vi "acq.Batch.vi"(6 "# Acq in":u16, 7 "DVR":T1, 8 "error in":errorcluster, 11 "cam in":refnum<class "camera.lvclass">) -> (0 "error out":errorcluster, 1 "PL":u16[][](array[numeric]), 2 "IL":u16[][](array[numeric]), 4 "acq time":dbl)   [LabVIEW 2020]
uses:
  c5544233-71f3-4b66-846b-1f2d698a5cd2.vi
  camera/camera.lvclass
  _controls/mode.ctl
  _controls/data.ref.ctl
  _controls/data.ctl
  _controls/state.ctl
  _controls/data.vars.ctl
  _controls/flip.ctl
  <vilib>/vision/Image Controls.llb/IMAQ Image.ctl
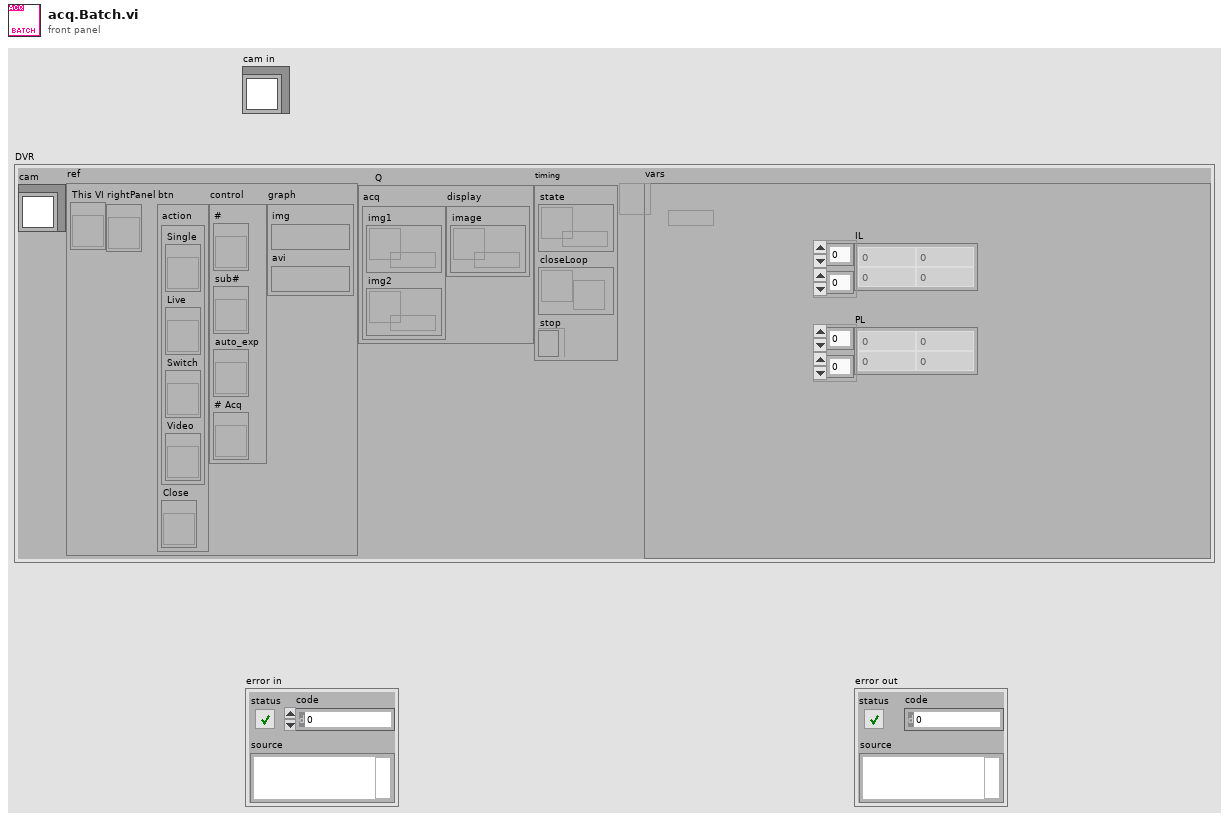
[diagram p1: front panel]
types:
  T1 = typedef "data.ctl" = cluster{"cam":refnum<class "camera.lvclass">, "ref":T2, "Q":cluster{"acq":cluster{"img1":refnum<queue>, "img2":refnum<queue>}, "display":cluster{"image":refnum<queue>}}, "timing":cluster{"state":refnum<queue>, "closeLoop":refnum<notifier>, "stop":refnum<k4>}, "vars":refnum<data-value>}
  T2 = typedef "data.ref.ctl" = cluster{"This VI":refnum<vi>, "rightPanel":refnum<vi>, "btn":cluster{"action":cluster{"Single":refnum<vi>, "Live":refnum<vi>, "Switch":refnum<vi>, "Video":refnum<vi>}, "Close":refnum<vi>}, "control":cluster{"#":refnum<vi>, "sub#":refnum<vi>, "auto_exp":refnum<vi>, "# Acq":refnum<vi>}, "graph":cluster{"img":T3, "avi":T3}}
  T3 = typedef "IMAQ Image.ctl" = refnum<image>
  T4 = typedef "mode.ctl" = enum16{"PL", "EL"}
  T5 = typedef "path.ctl" = cluster{"light":path, "name":string, "full":path}
  T6 = typedef "data.vars.ctl" = cluster{"save":cluster{"base_folder":cluster{"Folder":path, "tif":bool, "jpg":bool}, "module":string, "#":u32, "sub#":u8, "save.op":enum16{"Full", "Light"}, "same?":bool, "Shift":enum16{"Single", "Leapfrog"}, "jpg?":bool, "flip":T7}, "acq":cluster{"# Acq":u16, "rotate":bool, "FPS":dbl}, "calib.manual":cluster{"BG":cluster{"Image":u16[][], "enabled?":bool}, "FF":cluster{"Image":u16[][], "enabled?":bool}}}
  T7 = typedef "flip.ctl" = cluster{"x":bool, "y":bool}
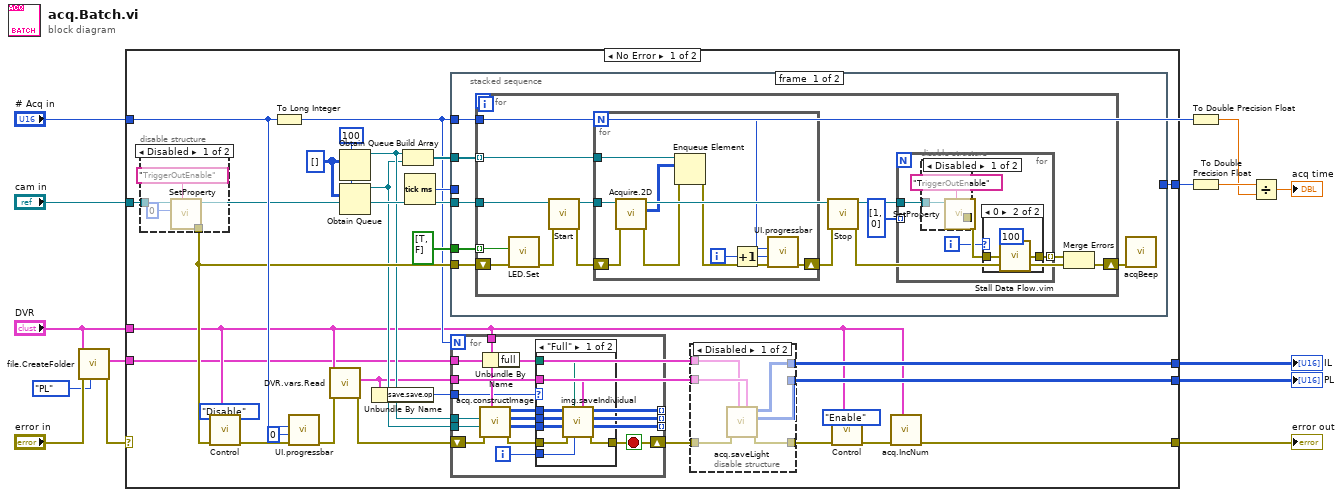
[diagram p0: block diagram]
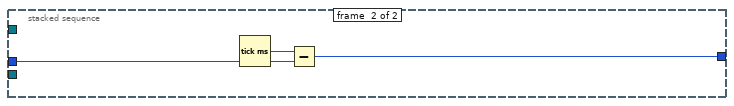
[diagram p6: hidden frame]
diagram:
  n1 = call "file.CreateFolder.vi"("mode"=mode."PL", "error in"="error in", "DVR"="DVR") -> ("error out"=w12:errorcluster, "path"=w9:T5)  [unwired: 7 in]
  n2 = case shown="No Error" w12 {
    selector: w12 -> [_ w118]
    tunnel: "cam in" -> [w31 _]
    tunnel: "# Acq in" -> [w42 _]
    tunnel: [w41 _] -> w13
    tunnel: [w27 w118] -> w2
    tunnel: "DVR" -> [w18 _]
    tunnel: [w25 _] -> w11
    tunnel: [w24 _] -> w10
    tunnel: w9 -> [w15 _]
    frame No Error {
      w36 = u16[][] [] ("buffer")
      w39 = 100 ("max queue size (-1, unlimited)")
      n3 = disable-structure shown="Disabled" {
        disable-tunnel: w31 -> [w52 _]
        disable-tunnel: [w51 _] -> w30
        frame Disabled {
          n4 = call-dynamic "SetProperty.vi"("Property"="TriggerOutEnable" ("pPrp"), "Value"=0 ("lValue"), "camera.nit in"=w52) -> ("error out"=w51:errorcluster)  [unwired: 8 in]
        }
        frame Enabled {
        }
      }
      n5 = call "Control.vi"("mode"=enum16{"Enable", "Disable"}."Disable", "DVR"=w18, "error in"=w30) -> ("error out"=w33:errorcluster)  [unwired: 8 in]
      n6 = To Long Integer(number=w42) -> (32bit integer=w19:i32)
      n7 = call "UI.progressbar.vi"("error in"=w33, "Value"=u8 0, "Maximum"=w42) -> ("error out"=w32:errorcluster)  [unwired: 8 in]
      n8 = call "DVR.vars.Read.vi"("error in"=w32, "DVR.state"=w18) -> ("error out"=w23:errorcluster, "vars"=w17:T6)  [unwired: 8 in]
      n9 = Obtain Queue(max queue size (-1, unlimited)=w39, element data type=w36) -> (queue out=w21:refnum<queue>)  [unwired: 3 in, 2 out]
      n10 = Obtain Queue(max queue size (-1, unlimited)=w39, element data type=w36) -> (queue out=w20:refnum<queue>)  [unwired: 3 in, 2 out]
      n11 = Unbundle By Name(w17) -> ("save.save.op"=w16:enum16{"Full", "Light"})
      n12 = Build Array(w21, w20) -> (w38:refnum<queue>[])
      n13 = Tick Count (ms)() -> (millisecond timer value=w37:u32)
      n14 = stacked-sequence {
        tunnel: bool[] [TRUE, FALSE] -> [w58 _]
        tunnel: w31 -> [w53 _]
        tunnel: w38 -> [w57 _]
        tunnel: w19 -> [w56 _]
        tunnel: w37 -> [_ w93]
        tunnel: [_ w92] -> w41
        tunnel: w30 -> [w55 _]
        frame #0 {
          n15 = for {
            tunnel: w56 -> [w66]
            shift-right: [w64] -> w54
            shift-left: w55 -> [w70]
            tunnel: w58 -> [w69] mode=indexing
            tunnel: w57 -> [w67] mode=indexing
            tunnel: w53 -> [w61]
            n16 = call "LED.Set.vi"("error in"=w70, "LED"=w69) -> ("error out"=w68:errorcluster)  [unwired: 9 in]
            n17 = call-dynamic "Start.vi"("error in"=w68, "camera in"=w61) -> ("error out"=w65:errorcluster)  [unwired: 9 in]
            n18 = for {
              N: w66 -> [w85]
              shift-right: [w83] -> w60
              shift-left: w65 -> [w89]
              tunnel: w61 -> [w90]
              tunnel: w67 -> [w91]
              i -> [w86]
              n19 = call-dynamic "Acquire.2D.vi"("error in"=w89, "camera.nit in"=w90) -> ("error out"=w88:errorcluster, "buffer"=w87:u16[][])  [unwired: 8 in]
              n20 = Enqueue Element(queue=w91, element=w87, error in (no error)=w88) -> (error out=w84:errorcluster)  [unwired: 1 in, 2 out]
              n21 = Increment(x=w86) -> (x+1=w82:i32)
              n22 = call "UI.progressbar.vi"("error in"=w84, "Value"=w82, "Maximum"=w85) -> ("error out"=w83:errorcluster)  [unwired: 8 in]
            }
            n23 = call-dynamic "Stop.vi"("error in"=w60, "camera.nit in"=w61) -> ("error out"=w59:errorcluster)  [unwired: 9 in]
            n24 = for {
              tunnel: w61 -> [w74]
              tunnel: [w72] -> w62 mode=indexing
              tunnel: i32[] [1, 0] ("0, 1") -> [_] mode=indexing
              i -> [w71]
              n25 = disable-structure shown="Disabled" {
                disable-tunnel: w74 -> [w77 _]
                disable-tunnel: [w76 _] -> w73
                frame Disabled {
                  n26 = call-dynamic "SetProperty.vi"("Property"="TriggerOutEnable" ("pPrp"), "camera.nit in"=w77) -> ("error out"=w76:errorcluster)  [unwired: 9 in]
                }
                frame Enabled {
                }
              }
              n27 = case shown="0" w71 {
                tunnel: w73 -> [w78 w81]
                tunnel: [w78 w80] -> w72
                frame Default {
                }
                frame 0 {
                  n28 = call "Stall Data Flow.vim"("value in"=w81, "milliseconds to wait"=u32 100) -> ("value out"=w80:errorcluster)  [unwired: 1 out]
                }
              }
            }
            n29 = Merge Errors(w62, w59) -> (w64:errorcluster)
          }
          n30 = call "acqBeep.vi"("error in"=w54) -> ()  [unwired: 10 in, 1 out]
        }
        frame #1 {
          n31 = Tick Count (ms)() -> (millisecond timer value=w94:u32)
          n32 = Subtract(x=w94, y=w93) -> (x-y=w92:u32)
        }
      }
      n33 = for {
        N: w19 -> [_]
        shift-right: [w98] -> w22
        shift-left: w23 -> [w106]
        tunnel: w20 -> [w107]
        tunnel: w21 -> [w108]
        tunnel: w18 -> [w105]
        tunnel: [w102] -> _ mode=indexing
        tunnel: [w101] -> _ mode=indexing
        tunnel: w17 -> [w100]
        tunnel: [w99] -> _ mode=indexing
        tunnel: w16 -> [w97]
        tunnel: w15 -> [w95]
        i -> [w103]
        stop <- w98 stop-if-true
        n34 = call "acq.constructImage.vi"("DVR"=w105, "error in"=w106, "queue2 in"=w107, "queue1 in"=w108) -> ("error out"=w104:errorcluster, "Dark"=w99:u16[][], "PL"=w101:u16[][], "Bright"=w102:u16[][])  [unwired: 4 in]
        n35 = Unbundle By Name(w95) -> ("full"=w96:path)
        n36 = case shown="\"Full\"" w97 {
          tunnel: w96 -> [w116 _]
          tunnel: w104 -> [w115 w117]
          tunnel: w103 -> [w114 _]
          tunnel: w102 -> [w113 _]
          tunnel: w101 -> [w112 _]
          tunnel: w100 -> [w111 _]
          tunnel: w99 -> [w110 _]
          tunnel: [w109 w117] -> w98
          frame "Full" {
            n37 = call "img.saveIndividual.vi"("vars"=w111, "loop"=w114, "path"=w116, "error in"=w115, "Dark"=w110, "PL"=w112, "Bright"=w113) -> ("error out"=w109:errorcluster)  [unwired: 4 in]
          }
          frame "Light" {
          }
        }
      }
      n38 = disable-structure shown="Disabled" {
        disable-tunnel: [w48 _] -> w26
        disable-tunnel: [w47 _] -> w25
        disable-tunnel: [w46 _] -> w24
        disable-tunnel: w22 -> [w45 _]
        disable-tunnel: w17 -> [w44 _]
        disable-tunnel: w15 -> [w43 _]
        frame Disabled {
          n39 = call "acq.saveLight.vi"("vars"=w44, "path"=w43, "error in"=w45) -> ("error out"=w48:errorcluster, "PL"=w46:u16[][], "IR"=w47:u16[][])  [unwired: 6 in]
        }
        frame Enabled {
        }
      }
      n40 = call "Control.vi"("mode"=enum16{"Enable", "Disable"}."Enable", "DVR"=w18, "error in"=w26) -> ("error out"=w29:errorcluster)  [unwired: 8 in]
      n41 = call "acq.IncNum.vi"("DVR in"=w18, "error in"=w29) -> ("error out"=w27:errorcluster)  [unwired: 9 in]
    }
    frame Error {
    }
  }
  "error out" <- w2
  "PL" <- w10
  "IL" <- w11
  n42 = To Double Precision Float(number="# Acq in") -> (double precision float=w4:dbl)
  n43 = To Double Precision Float(number=w13) -> (double precision float=w6:dbl)
  n44 = Divide(x=w6, y=w4) -> (x/y=→"acq time":dbl)
